vi "triple Lockin SCTL.vi"(6 "phases valid":bool, 7 "reset":bool, 8 "phases in":fxp<+,26,1>[](array[numeric])=[0.0, 0.0, 0.0], 9 "AI Valid":bool, 10 "AI in":fxp<+/-,16,1>, 11 "param":T2={"harmonic"=[63.99993896484375, 63.99993896484375, 63.99993896484375], "LP1 coeffs"=[-1025014616, 2098093632, 165702, -1053286467, 2126356551, 167935, -1025014616, 2098093632, 165702, -1053286467, 2126356551, 167935, -1025014616, 2098093632, 165702, -1053286467, 2126356551, 167935], "scope on"=FALSE, "scope channel"=0, "scope signal"=0}) -> (1 "magnitude out":fxp<+,16,1>[](array[numeric]), 2 "phase block valid":bool, 3 "unwrapped phases out":fxp<+,26,12>[](array[numeric]))   [LabVIEW 2018, in "SCTL.lvlib"]
uses:
  SCTL.lvlib
  param-sctl-lockin.ctl
  param-sctl-pll.ctl
  <vilib>/rvi/FXPMathLib/FxpSinAndCos/subVIs/nifxpmath_SinAndCos_SimConfig.ctl
  <vilib>/rvi/FXPMathLib/FxpRectToPolar/subVIs/nifxpmath_RectToPolar_SimConfig.ctl
  <vilib>/rvi/FXPMathLib/FxpSinAndCos/simVIs/DllFxpSinAndCosTemp_sub.vi
  <vilib>/rvi/FXPMathLib/FxpRectToPolar/simVIs/DllFxpRectToPolarTemp_sub.vi
  <vilib>/rvi/FXPMathLib/FxpMul/XNode/nifxpmath_Multiplier.xnode
  <vilib>/rvi/FXPMathLib/FxpSinAndCos/XNode/nifxpmath_SinAndCos.xnode
  <vilib>/rvi/FXPMathLib/FxpRectToPolar/XNode/nifxpmath_RectToPolar.xnode
  <vilib>/rvi/FXPMathLib/FxpSub/XNode/nifxpmath_Sub.xnode
  <vilib>/rvi/FXPMathLib/FxpAdd/XNode/nifxpmath_Add.xnode
  <vilib>/rvi/FXPMathLib/sim/FxpSim.dll
panel:
  in  "param pll (for type)":T1={"base freq (Hz)"=[20123.0, 20123.0, 20123.0], "P gain"=[1234.0, 1234.0, 1234.0], "I gain"=[1.0, 1.0, 1.0], "LP1 coeffs"=[-1025014616, 2098093632, 165702, -1053286467, 2126356551, 167935, -1025014616, 2098093632, 165702, -1053286467, 2126356551, 167935, -1025014616, 2098093632, 165702, -1053286467, 2126356551, 167935], "scope on"=FALSE, "scope channel"=0, "scope signal"=0, "notch coeff"=[-1025014616, 2098093632, 165702, -1053286467, 2126356551, 167935, -1025014616, 2098093632, 165702]}
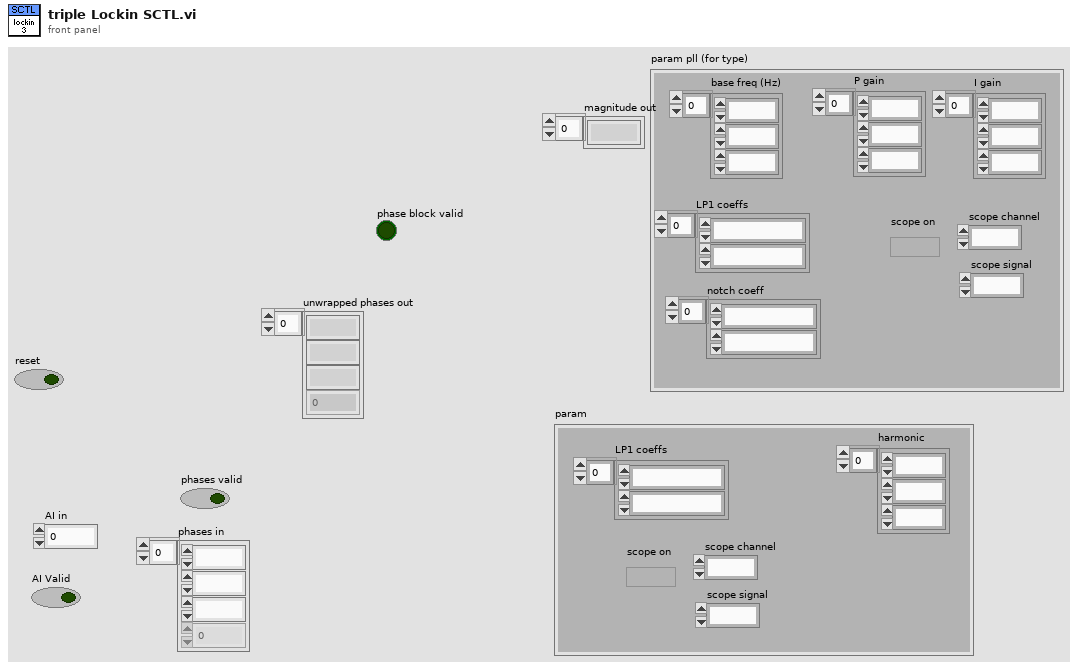
[diagram p1: front panel]
types:
  T1 = typedef "SCTL.lvlib/param-sctl-pll.ctl" = cluster{"base freq (Hz)":fxp<+,17,17>[], "P gain":fxp<+,14,14>[], "I gain":fxp<+,20,6>[], "LP1 coeffs":i32[], "scope on":bool, "scope channel":u8, "scope signal":u8, "notch coeff":i32[]}
  T2 = typedef "param-sctl-lockin.ctl" = cluster{"harmonic":fxp<+,20,6>[], "LP1 coeffs":i32[], "scope on":bool, "scope channel":u8, "scope signal":u8}
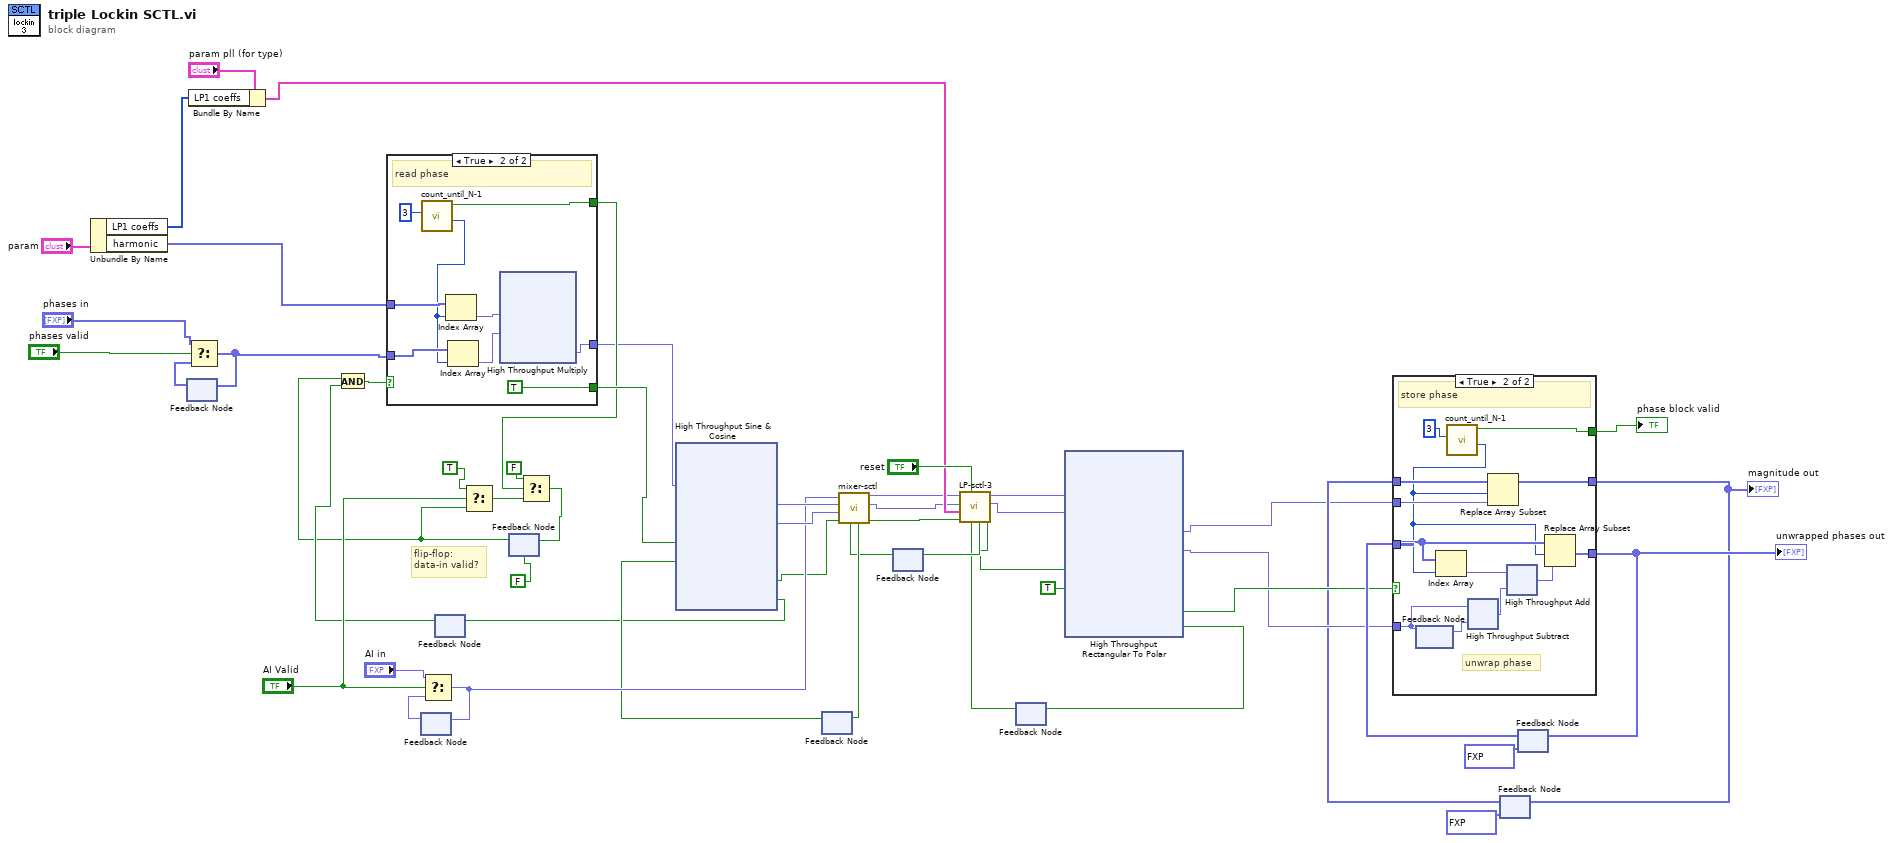
[diagram p0: block diagram]
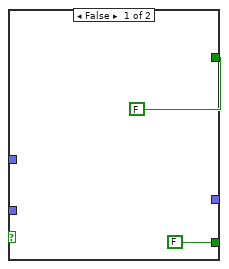
[diagram p2: hidden frame]
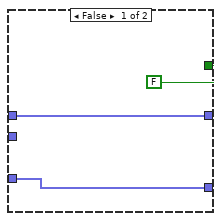
[diagram p3: hidden frame]
diagram:
  # "flip-flop:\ndata-in valid?"
  n1 = Unbundle By Name("param") -> ("LP1 coeffs"=w15:i32[], "harmonic"=w18:fxp<+,20,6>[])
  n2 = feedback #1() -> (w23:fxp<+,26,1>[])  [unwired: 1 in]
  n3 = Bundle By Name(cluster="param pll (for type)", "LP1 coeffs"=w15) -> (w14:T1)
  n4 = Select(t="phases in", s="phases valid", f=w23) -> (s? t:f=w20:fxp<+,26,1>[])
  n5 = feedback-in #1(w20) -> ()
  n6 = feedback #2() -> (w35:fxp<+/-,16,1>)  [unwired: 1 in]
  n7 = Select(t="AI in", s="AI Valid", f=w35) -> (s? t:f=w46:fxp<+/-,16,1>)
  n8 = feedback-in #2(w46) -> ()
  n9 = feedback #3() -> (w28:bool)  [unwired: 1 in]
  n10 = feedback #4(FALSE) -> (w25:bool)
  n11 = And(x=w25, y=w28) -> (x .and. y?=w27:bool)
  n12 = case shown="True" w27 {
    tunnel: [FALSE w56] -> w32
    tunnel: [FALSE ("input valid") TRUE ("input valid")] -> w36
    tunnel: w20 -> [_ w62]
    tunnel: w18 -> [_ w61]
    tunnel: [_ w58] -> w17
    frame False {
    }
    frame True {
      # "read phase"
      n13 = call "count_until_N-1.vi"("N"=u8 3) -> ("counter"=w55:u8, "turn around !"=w56:bool)  [unwired: 9 in]
      n14 = Index Array(array=w61, index=w55) -> (element=w60:fxp<+,20,6>)
      n15 = Index Array(array=w62, index=w55) -> (element=w59:fxp<+,26,1>)
      n16 = xnode ("High Throughput Multiply")("x"=w60, "y"=w59) -> ("x*y"=w58:fxp<+,26,1>)
    }
  }
  n17 = Select(t=TRUE ("input valid"), s="AI Valid", f=w25) -> (s? t:f=w31:bool)
  n18 = Select(t=FALSE ("input valid"), s=w32, f=w31) -> (s? t:f=w29:bool)
  n19 = feedback-in #4(w29) -> ()
  n20 = feedback #5() -> (w45:bool)  [unwired: 1 in]
  n21 = xnode ("High Throughput Sine & Cosine")("x (pi)"=w17, "input valid"=w36, "ready for output (T)"=w45) -> ("sin(x)"=w52:fxp<+/-,16,2>, "cos(x)"=w51:fxp<+/-,16,2>, "output valid"=w38:bool, "ready for input"=w39:bool)
  n22 = feedback-in #3(w39) -> ()
  n23 = feedback #6() -> (w48:bool)  [unwired: 1 in]
  n24 = call "mixer-sctl.vi"("Ready For Output"=w48, "Input Valid"=w38, "cos"=w51, "sin"=w52, "AI"=w46) -> ("Output Valid"=w43:bool, "Y"=w8:fxp<+/-,20,2>, "X"=w9:fxp<+/-,20,2>, "Ready For Input"=w50:bool)  [unwired: 3 in]
  n25 = feedback-in #5(w50) -> ()
  n26 = feedback #7() -> (w47:bool)  [unwired: 1 in]
  n27 = call "LP-sctl-3.vi"("Ready For Output"=w47, "reset"="reset", "Input Valid"=w43, "param"=w14, "Y in"=w8, "X in"=w9) -> ("Output Valid"=w13:bool, "Y out"=w6:fxp<+/-,16,1>, "X out"=w7:fxp<+/-,16,1>, "Ready For Input"=w49:bool)  [unwired: 2 in]
  n28 = feedback-in #6(w49) -> ()
  n29 = xnode "High Throughput Rectangular To Polar"("x"=w7, "y"=w6, "input valid"=w13, "ready for output (T)"=TRUE) -> ("magnitude"=w1:fxp<+,16,1>, "phase (pi)"=w5:fxp<+/-,16,2>, "output valid"=w10:bool, "ready for input"=w11:bool)
  n30 = feedback-in #7(w11) -> ()
  n31 = feedback #8(fxp<+,16,1>[] [0.0, 0.0, 0.0] ("Array")) -> (w3:fxp<+,16,1>[])
  n32 = feedback #9(fxp<+,26,12>[] [0.0, 0.0, 0.0] ("Array")) -> (w24:fxp<+,26,12>[])
  n33 = case shown="True" w10 {
    tunnel: [w65 w79] -> w40
    tunnel: [FALSE w67] -> w42
    tunnel: w24 -> [w65 w75]
    tunnel: w5 -> [_ w72]
    tunnel: w3 -> [w64 w78]
    tunnel: [w64 w77] -> w2
    tunnel: w1 -> [_ w76]
    frame False {
    }
    frame True {
      # "unwrap phase"
      # "store phase"
      n34 = feedback-in #10(w72) -> ()
      n35 = feedback #10() -> (w73:fxp<+/-,16,2>)  [unwired: 1 in]
      n36 = call "count_until_N-1.vi"("N"=u8 3) -> ("counter"=w68:u8, "turn around !"=w67:bool)  [unwired: 9 in]
      n37 = Index Array(array=w75, index=w68) -> (element=w71:fxp<+,26,12>)
      n38 = xnode "High Throughput Subtract"("x"=w72, "y"=w73) -> ("x-y"=w70:fxp<+/-,16,2>)
      n39 = Replace Array Subset(array=w78, new element=w76, index=w68) -> (w77:fxp<+,16,1>[])
      n40 = xnode ("High Throughput Add")("x"=w71, "y"=w70) -> ("x+y"=w74:fxp<+,26,12>)
      n41 = Replace Array Subset(array=w75, new element=w74, index=w68) -> (w79:fxp<+,26,12>[])
    }
  }
  "unwrapped phases out" <- w40
  "phase block valid" <- w42
  "magnitude out" <- w2
  n42 = feedback-in #8(w2) -> ()
  n43 = feedback-in #9(w40) -> ()
